vi "Create TX resource Instance.vi"(10 "instance":u8, 11 "niUSRP Tx DSP v2 FPGA in":refnum<class "niUSRP Tx DSP v2 FPGA.lvclass">) -> (0 "TxDspEnabled":u64, 2 "address space collection":refnum<class "Address Space Collection.lvclass">, 3 "niUSRP Tx DSP v2 FPGA out":refnum<class "niUSRP Tx DSP v2 FPGA.lvclass">)   [LabVIEW 2025, in "niUSRP Tx DSP v2 FPGA.lvclass"]
uses:
  niUSRP Tx DSP v2 FPGA.lvclass
  <instrlib>/_niInstr/Instruction Framework/v1/FPGA/Interfaces/Address Space Collection/Address Space Collection.lvclass
  <instrlib>/_niInstr/DSP Control/Common/v2/FPGA/Resampling/Harness Type.ctl
  <instrlib>/_niInstr/DSP Control/Common/v2/FPGA/Equalization/Registers/Equalization Filter Type.ctl
  <instrlib>/_niInstr/Instruction Framework/v1/FPGA/Collection Builder/Collection Builder.lvclass
  <instrlib>/_niInstr/DSP Control/Interface/v1/FPGA/niInstr DSP Control Interface v1 FPGA.lvlib
  <instrlib>/_niInstr/Basic Elements/v1/FPGA/niInstr Basic Elements v1 FPGA.lvlib
  <instrlib>/_niInstr/DSP Control/Common/v2/FPGA/Equalization/Registers/Equalization Registers.lvclass
  <instrlib>/_niInstr/DSP Control/Common/v2/FPGA/Resampling/Resampler Harness.lvclass
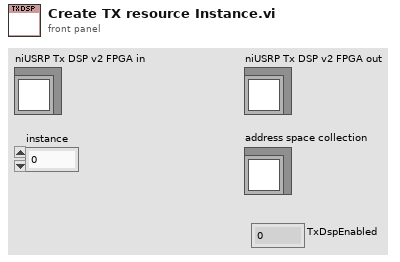
[diagram p1: front panel]
types:
  T1 = typedef "niInstr DSP Control Common v2 FPGA.lvlib/Equalization Registers.lvclass/Equalization Filter Type.ctl" = enum8{"Undefined", "Single", "Complex", "Matrix"}
  T2 = typedef "niInstr DSP Control Common v2 FPGA.lvlib/Resampler Harness.lvclass/Harness Type.ctl" = enum16{"None", "Integer Linear", "Integer List", "Integer-Exponential", "Fixed Rational", "Fractional (16-bit Delay)", "Fractional (18-bit Delay)", "Rational List", "External", "External and Fractional"}
  T3 = typedef "niInstr Address Space Collection Builder v1 FPGA.lvlib/Parent Metadata.ctl" = cluster{"UID":u16, "version":u16, "oldest compatible version":u16}
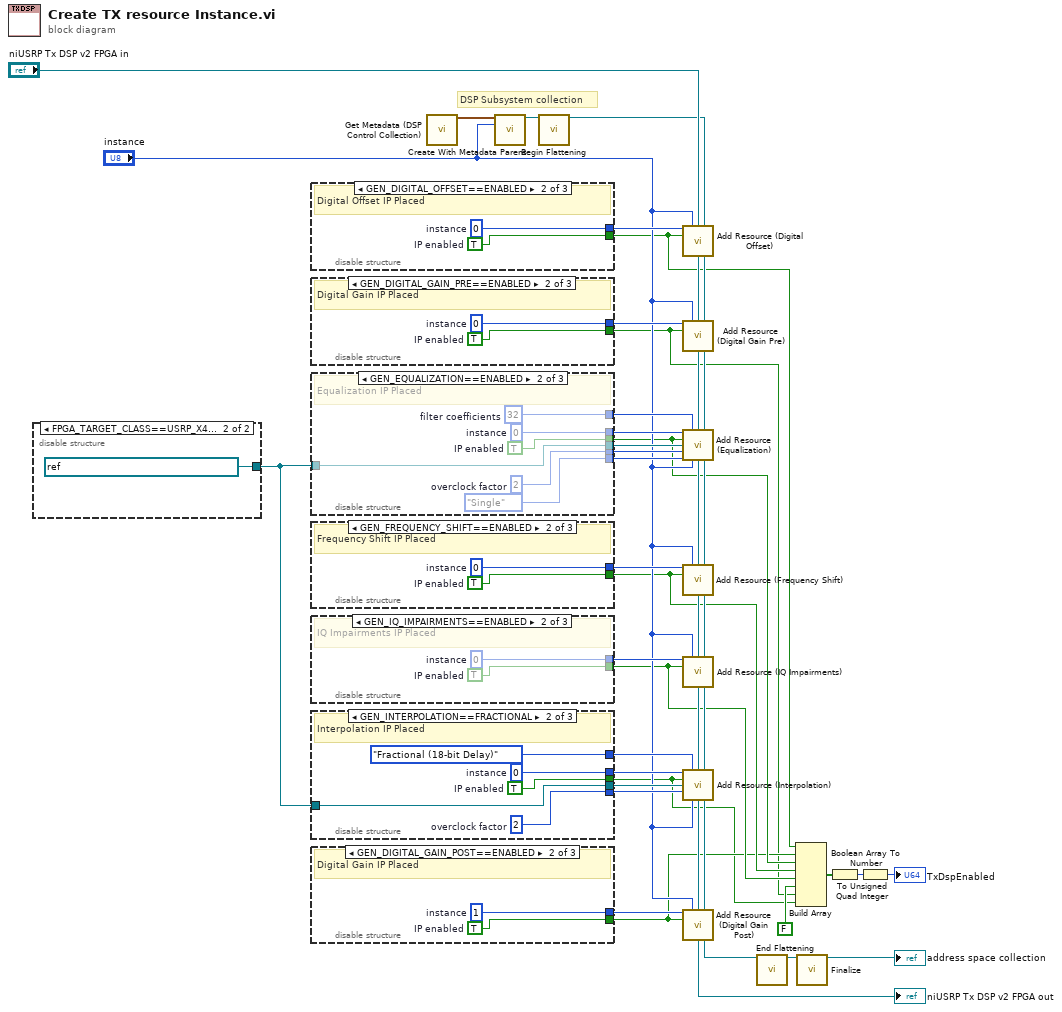
[diagram p0: block diagram]
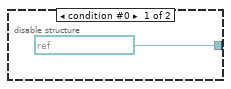
[diagram p2: hidden frame]
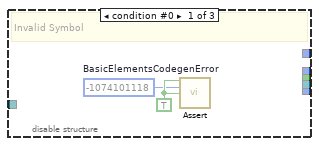
[diagram p3: hidden frame]
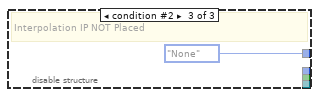
[diagram p4: hidden frame]
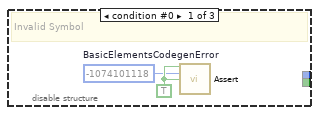
[diagram p5: hidden frame]
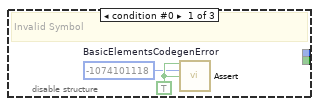
[diagram p7: hidden frame]
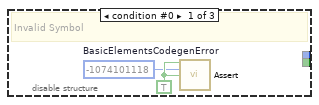
[diagram p9: hidden frame]
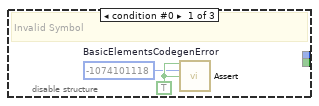
[diagram p11: hidden frame]
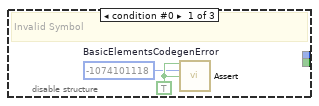
[diagram p13: hidden frame]
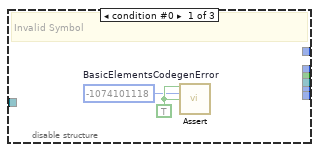
[diagram p15: hidden frame]
diagram:
  # "DSP Subsystem collection"
  n1 = disable-structure shown="FPGA_TARGET_CLASS==USRP_X410||FPGA_TARGET_CLASS==USRP_X410__EMBEDDED____UNSUPPORTED" {
    disable-tunnel: [refnum<k21> "Data Clock x2" ("clock x2") refnum<k21> "Daughterboard 0\\Data Clock x2" ("clock x2")] -> w47
    frame condition #0 {
    }
    frame condition #1 (active) {
    }
  }
  n2 = disable-structure shown="GEN_DIGITAL_OFFSET==ENABLED" {
    disable-tunnel: [_ w53 _] -> w26
    disable-tunnel: [_ w52 _] -> w8
    frame condition #0 {
      w51 = TRUE ("assert")
      w50 = -1074101118  # BasicElementsCodegenError
      # "Invalid Symbol"
      n3 = call <instrlib>:"Assert.vi"("assert"=w51, "error code"=w50, "enable show error"=w51) -> ()  [unwired: 13 in]
    }
    frame condition #1 (active) {
      w52 = TRUE  # IP enabled
      w53 = u8 0  # instance
      # "Digital Offset IP Placed"
    }
    frame condition #2 {
      # "Digital Offset IP NOT Placed"
    }
  }
  n4 = disable-structure shown="GEN_DIGITAL_GAIN_PRE==ENABLED" {
    disable-tunnel: [_ w57 _] -> w27
    disable-tunnel: [_ w56 _] -> w2
    frame condition #0 {
      w55 = TRUE ("assert")
      w54 = -1074101118  # BasicElementsCodegenError
      # "Invalid Symbol"
      n5 = call <instrlib>:"Assert.vi"("assert"=w55, "error code"=w54, "enable show error"=w55) -> ()  [unwired: 13 in]
    }
    frame condition #1 (active) {
      w56 = TRUE  # IP enabled
      w57 = u8 0  # instance
      # "Digital Gain IP Placed"
    }
    frame condition #2 {
      # "Digital Gain IP NOT Placed"
    }
  }
  n6 = disable-structure shown="GEN_EQUALIZATION==ENABLED" {
    disable-tunnel: [_ w65 _] -> w18
    disable-tunnel: [_ w64 _] -> w7
    disable-tunnel: [_ w63 _] -> w17
    disable-tunnel: [_ w60 _] -> w19
    disable-tunnel: [_ w62 _] -> w20
    disable-tunnel: [_ Equalization_Filter_Type."Single" ("filter type") _] -> w46
    disable-tunnel: w47 -> [_ w60 _]
    frame condition #0 {
      w59 = TRUE ("assert")
      w58 = -1074101118  # BasicElementsCodegenError
      # "Invalid Symbol"
      n7 = call <instrlib>:"Assert.vi"("assert"=w59, "error code"=w58, "enable show error"=w59) -> ()  [unwired: 13 in]
    }
    frame condition #1 {
      w62 = u8 32  # filter coefficients
      w63 = u8 2  # overclock factor
      w64 = TRUE  # IP enabled
      w65 = u8 0  # instance
      # "Equalization IP Placed"
    }
    frame condition #2 (active) {
      # "Equalization IP NOT Placed"
    }
  }
  n8 = disable-structure shown="GEN_FREQUENCY_SHIFT==ENABLED" {
    disable-tunnel: [_ w69 _] -> w28
    disable-tunnel: [_ w68 _] -> w6
    frame condition #0 {
      w67 = TRUE ("assert")
      w66 = -1074101118  # BasicElementsCodegenError
      # "Invalid Symbol"
      n9 = call <instrlib>:"Assert.vi"("assert"=w67, "error code"=w66, "enable show error"=w67) -> ()  [unwired: 13 in]
    }
    frame condition #1 (active) {
      w68 = TRUE  # IP enabled
      w69 = u8 0  # instance
      # "Frequency Shift IP Placed"
    }
    frame condition #2 {
      # "Frequency Shift IP NOT Placed"
    }
  }
  n10 = disable-structure shown="GEN_IQ_IMPAIRMENTS==ENABLED" {
    disable-tunnel: [_ w73 _] -> w29
    disable-tunnel: [_ w72 _] -> w5
    frame condition #0 {
      w71 = TRUE ("assert")
      w70 = -1074101118  # BasicElementsCodegenError
      # "Invalid Symbol"
      n11 = call <instrlib>:"Assert.vi"("assert"=w71, "error code"=w70, "enable show error"=w71) -> ()  [unwired: 13 in]
    }
    frame condition #1 {
      w72 = TRUE  # IP enabled
      w73 = u8 0  # instance
      # "IQ Impairments IP Placed"
    }
    frame condition #2 (active) {
      # "IQ Impairments IP NOT Placed"
    }
  }
  n12 = disable-structure shown="GEN_INTERPOLATION==FRACTIONAL" {
    disable-tunnel: [_ w80 _] -> w38
    disable-tunnel: [_ w79 _] -> w1
    disable-tunnel: [_ w78 _] -> w40
    disable-tunnel: [_ w76 _] -> w39
    disable-tunnel: [_ Harness_Type."Fractional (18-bit Delay)" ("harness type") Harness_Type."None" ("harness type")] -> w37
    disable-tunnel: w47 -> [_ w76 _]
    frame condition #0 {
      w75 = TRUE ("assert")
      w74 = -1074101118  # BasicElementsCodegenError
      # "Invalid Symbol"
      n13 = call <instrlib>:"Assert.vi"("assert"=w75, "error code"=w74, "enable show error"=w75) -> ()  [unwired: 13 in]
    }
    frame condition #1 (active) {
      w78 = u8 2  # overclock factor
      w79 = TRUE  # IP enabled
      w80 = u8 0  # instance
      # "Interpolation IP Placed"
    }
    frame condition #2 {
      # "Interpolation IP NOT Placed"
    }
  }
  n14 = disable-structure shown="GEN_DIGITAL_GAIN_POST==ENABLED" {
    disable-tunnel: [_ w85 _] -> w32
    disable-tunnel: [_ w84 _] -> w4
    frame condition #0 {
      w83 = TRUE ("assert")
      w82 = -1074101118  # BasicElementsCodegenError
      # "Invalid Symbol"
      n15 = call <instrlib>:"Assert.vi"("assert"=w83, "error code"=w82, "enable show error"=w83) -> ()  [unwired: 13 in]
    }
    frame condition #1 (active) {
      w84 = TRUE  # IP enabled
      w85 = u8 1  # instance
      # "Digital Gain IP Placed"
    }
    frame condition #2 {
      # "Digital Gain IP NOT Placed"
    }
  }
  n16 = call <instrlib>:"Get Metadata (DSP Control Collection).vi"() -> ("parent metadata"=w43:T3)  [unwired: 15 in]
  n17 = call <instrlib>:"Create With Metadata Parent.vi"("parent metadata"=w43, "instance (0)"="instance") -> ("collection builder"=w41:refnum<class "Collection Builder.lvclass">)  [unwired: 13 in]
  n18 = call <instrlib>:"Begin Flattening.vi"("collection builder in"=w41) -> ("collection builder out"=w42:refnum<class "Collection Builder.lvclass">)  [unwired: 14 in]
  n19 = call-dynamic "Add Resource (Digital Offset).vi"("instance"=w26, "channel"="instance", "gen in"="niUSRP Tx DSP v2 FPGA in", "collection builder in"=w42, "IP enabled"=w8) -> ("gen out"=w16:refnum<class "niUSRP Tx DSP v2 FPGA.lvclass">, "collection builder out"=w23:refnum<class "Collection Builder.lvclass">)  [unwired: 9 in]
  n20 = call-dynamic "Add Resource (Digital Gain Pre).vi"("instance"=w27, "channel"="instance", "gen in"=w16, "collection builder in"=w23, "IP enabled"=w2) -> ("gen out"=w21:refnum<class "niUSRP Tx DSP v2 FPGA.lvclass">, "collection builder out"=w22:refnum<class "Collection Builder.lvclass">)  [unwired: 9 in]
  n21 = call-dynamic "Add Resource (Equalization).vi"("instance"=w18, "number of filter coefficients"=w20, "gen in"=w21, "collection builder in"=w22, "IP enabled"=w7, "overclock"=w19, "overclock factor"=w17, "filter type"=w46, "channel"="instance") -> ("gen out"=w24:refnum<class "niUSRP Tx DSP v2 FPGA.lvclass">, "collection builder out"=w25:refnum<class "Collection Builder.lvclass">)  [unwired: 5 in]
  n22 = call-dynamic "Add Resource (Frequency Shift).vi"("instance"=w28, "channel"="instance", "gen in"=w24, "collection builder in"=w25, "IP enabled"=w6) -> ("gen out"=w30:refnum<class "niUSRP Tx DSP v2 FPGA.lvclass">, "collection builder out"=w31:refnum<class "Collection Builder.lvclass">)  [unwired: 9 in]
  n23 = call-dynamic "Add Resource (IQ Impairments).vi"("instance"=w29, "channel"="instance", "gen in"=w30, "collection builder in"=w31, "IP enabled"=w5) -> ("gen out"=w35:refnum<class "niUSRP Tx DSP v2 FPGA.lvclass">, "collection builder out"=w36:refnum<class "Collection Builder.lvclass">)  [unwired: 9 in]
  n24 = call-dynamic "Add Resource (Interpolation).vi"("instance"=w38, "harness type"=w37, "gen in"=w35, "collection builder in"=w36, "IP enabled"=w1, "overclock"=w39, "overclock factor"=w40, "channel"="instance") -> ("gen out"=w33:refnum<class "niUSRP Tx DSP v2 FPGA.lvclass">, "collection builder out"=w34:refnum<class "Collection Builder.lvclass">)  [unwired: 6 in]
  n25 = call-dynamic "Add Resource (Digital Gain Post).vi"("instance"=w32, "channel"="instance", "gen in"=w33, "collection builder in"=w34, "IP enabled"=w4) -> ("gen out"=→"niUSRP Tx DSP v2 FPGA out":refnum<class "niUSRP Tx DSP v2 FPGA.lvclass">, "collection builder out"=w15:refnum<class "Collection Builder.lvclass">)  [unwired: 9 in]
  n26 = call <instrlib>:"End Flattening.vi"("collection builder in"=w15) -> ("collection builder out"=w14:refnum<class "Collection Builder.lvclass">)  [unwired: 14 in]
  n27 = Build Array(w8, w4, w7, w6, w5, FALSE, w2, w1) -> (w11:bool[])
  n28 = call <instrlib>:"Finalize.vi"("collection builder in"=w14) -> ("address space collection"=→"address space collection":refnum<class "Address Space Collection.lvclass">)  [unwired: 14 in]
  n29 = Boolean Array To Number(Boolean array=w11) -> (number=w10:u8)
  n30 = To Unsigned Quad Integer(1:w10) -> (0:→"TxDspEnabled":u64)
